vi "mathexperiments.vi"() -> ()   [LabVIEW 2018]
uses:
  <vilib>/Analysis/4window.llb/windowTd.ctl
  <vilib>/measure/maspectr.llb/FFT Power Spectrum and PSD for 1 Chan.vi
  <vilib>/measure/NI_MABase.lvlib
  <vilib>/measure/NI_MAPro.lvlib
  <vilib>/Analysis/NI_AALPro.lvlib
  <vilib>/rtlsdr/rtlsdr.lvlib
panel:
  out "Waveform Graph 3":waveform(dbl)(graph)
  out "Waveform Graph 2":waveform(dbl)(graph)
  in  "sampling info":cluster{"Fs":dbl, "#s":dbl}={"Fs"=1000.0, "#s"=1000.0} {"Fs" format="%.2p"}
  out "size(s)":i32
  out "dt":dbl
  in  "dB On (F)":bool
  in  "stop":bool
  in  "window":T1=1 items=["Rectangle"=0, "Hanning"=1, "Hamming"=2, "Blackman-Harris"=3, "Exact Blackman"=4, "Blackman"=5, "Flat Top"=6, "4 Term B-Harris "=7, "7 Term B-Harris"=8, "Low Sidelobe"=9, "Blackman Nuttall"=11, "Triangle"=30, "Bartlett-Hanning"=31, "Bohman"=32, "Parzen"=33, "Welch"=34, "Kaiser"=60, "Dolph-Chebyshev"=61, "Gaussian"=62]
  out "Waveform Graph":cluster{"f0":dbl, "df":dbl, "magnitude":dbl[]}(graph)
  in  "Amplitude":dbl
  in  "Frequency (Hz)":dbl(knob) scale=0.0..500.0
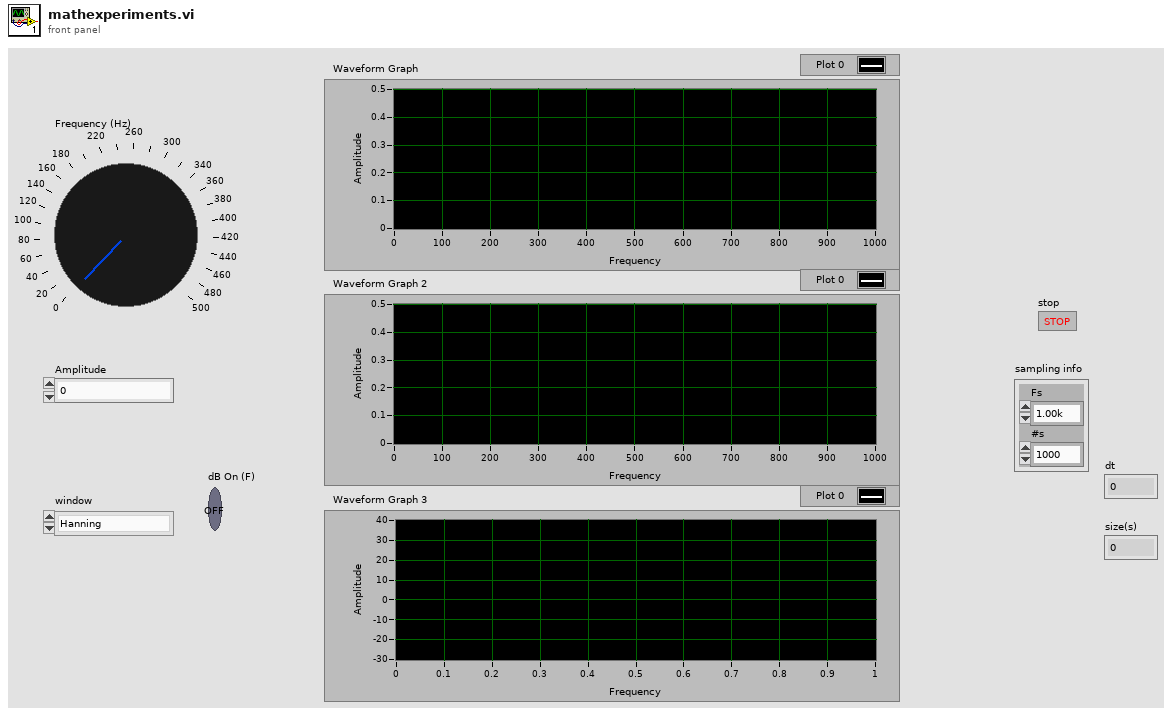
[diagram p1: front panel]
types:
  T1 = typedef "NI_AALPro.lvlib/windowTd.ctl" = u32
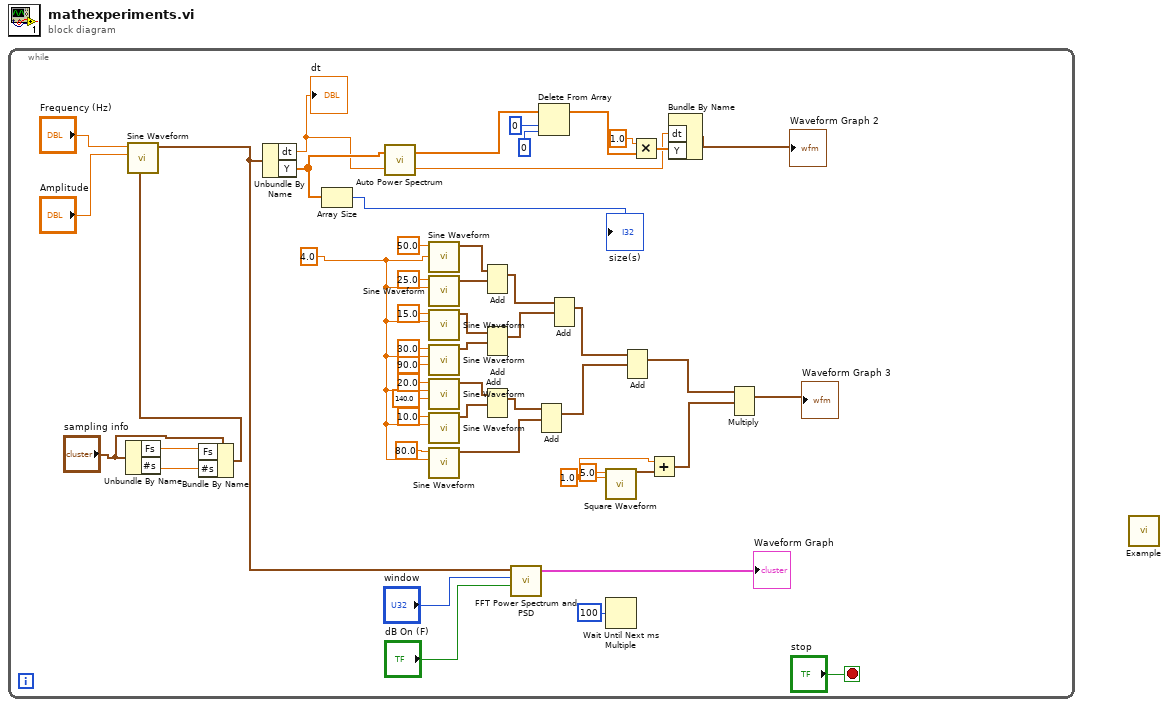
[diagram p0: block diagram]
diagram:
  n1 = while {
    stop <- "stop" stop-if-true
    w20 = 1.0 ("amplitude")
    w7 = 4.0
    n2 = Unbundle By Name("sampling info") -> ("Fs"=w35:dbl, "#s"=w3:dbl)
    n3 = Bundle By Name(cluster="sampling info", "Fs"=w35, "#s"=w3) -> (w34:cluster{"Fs":dbl, "#s":dbl})
    n4 = call <vilib>:"Sine Waveform.vi"("sampling info"=w34, "amplitude"="Amplitude", "frequency"="Frequency (Hz)") -> ("signal out"=w32:waveform(dbl))  [unwired: 7 in, 1 out]
    n5 = Unbundle By Name(w32) -> ("dt"=w2:dbl, "Y"=w40:dbl[])
    "dt" <- w2
    n6 = Array Size(array=w40) -> (size(s)=→"size(s)":i32)
    n7 = call <vilib>:"Auto Power Spectrum.vi"("dt"=w2, "Signal (V)"=w40) -> ("df"=w1:dbl, "Power Spectrum (V^2 rms)"=w37:dbl[])
    n8 = call <vilib>:"Sine Waveform.vi"("amplitude"=w7, "frequency"=50.0) -> ("signal out"=w14:waveform(dbl))  [unwired: 8 in, 1 out]
    n9 = call <vilib>:"Sine Waveform.vi"("amplitude"=w7, "frequency"=25.0) -> ("signal out"=w15:waveform(dbl))  [unwired: 8 in, 1 out]
    n10 = call <vilib>:"Sine Waveform.vi"("amplitude"=w7, "frequency"=15.0) -> ("signal out"=w19:waveform(dbl))  [unwired: 8 in, 1 out]
    n11 = call <vilib>:"Sine Waveform.vi"("phase"=90.0, "amplitude"=w7, "frequency"=30.0) -> ("signal out"=w18:waveform(dbl))  [unwired: 7 in, 1 out]
    n12 = call <vilib>:"Sine Waveform.vi"("phase"=140.0, "amplitude"=w7, "frequency"=20.0) -> ("signal out"=w17:waveform(dbl))  [unwired: 7 in, 1 out]
    n13 = call <vilib>:"Sine Waveform.vi"("amplitude"=w7, "frequency"=10.0) -> ("signal out"=w16:waveform(dbl))  [unwired: 8 in, 1 out]
    n14 = call <vilib>:"Sine Waveform.vi"("amplitude"=w7, "frequency"=80.0) -> ("signal out"=w12:waveform(dbl))  [unwired: 8 in, 1 out]
    n15 = Add(1:w15, 2:w14) -> (0:w11:waveform(dbl))  [unwired: 1 in, 1 out]
    n16 = Add(1:w18, 2:w19) -> (0:w10:waveform(dbl))  [unwired: 1 in, 1 out]
    n17 = Add(1:w16, 2:w17) -> (0:w13:waveform(dbl))  [unwired: 1 in, 1 out]
    n18 = call-poly <vilib>:"FFT Power Spectrum and PSD.vi"("dB On (F)"="dB On (F)", "window"="window", "time signal"=w32) -> ("Power Spectrum / PSD"=→"Waveform Graph":cluster{"f0":dbl, "df":dbl, "magnitude":dbl[]})  [unwired: 5 in, 3 out]
    n19 = Add(1:w12, 2:w13) -> (0:w8:waveform(dbl))  [unwired: 1 in, 1 out]
    n20 = Delete From Array(array=w37, length=0, index=0) -> (array with subset deleted=w44:dbl[])  [unwired: 1 out]
    n21 = Add(1:w10, 2:w11) -> (0:w9:waveform(dbl))  [unwired: 1 in, 1 out]
    n22 = call <vilib>:"Square Waveform.vi"("amplitude"=w20, "frequency"=5.0) -> ("signal out"=w21:waveform(dbl))  [unwired: 8 in, 1 out]
    n23 = Wait Until Next ms Multiple(millisecond multiple=u32 100) -> ()  [unwired: 1 out]
    n24 = Add(1:w8, 2:w9) -> (0:w6:waveform(dbl))  [unwired: 1 in, 1 out]
    n25 = Multiply(x=1.0, y=w44) -> (x*y=w41:dbl[])
    n26 = Add(x=w20, y=w21) -> (x+y=w5:waveform(dbl))
    n27 = Bundle By Name("dt"=w1, "Y"=w41) -> (→"Waveform Graph 2":waveform(dbl))  [unwired: 1 in]
    n28 = Multiply(1:w5, 2:w6) -> (0:→"Waveform Graph 3":waveform(dbl))  [unwired: 1 in, 1 out]
  }
  n29 = call <vilib>:"Example.vi"() -> ()  [unwired: 12 in]
